vi "亮度变换.vi"(11 "in":dbl) -> (3 "out":dbl)   [LabVIEW 2012]
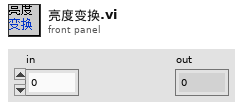
[diagram p1: front panel]
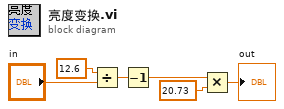
[diagram p0: block diagram]
diagram:
  n1 = Divide(x=12.6 ("y"), y="in") -> (x/y=w1:dbl)
  n2 = Decrement(x=w1) -> (x-1=w6:dbl)
  n3 = Multiply(x=w6, y=20.73) -> (x*y=→"out":dbl)
